vi "Utilisation des boucles.vi"() -> ()   [LabVIEW 2017]
panel:
  in  "V end":dbl format="%#_13g"
  in  "V0":dbl format="%#_13g"
  out "Waveform Graph 2":dbl[](graph)
  in  "Step":dbl format="%#_13g"
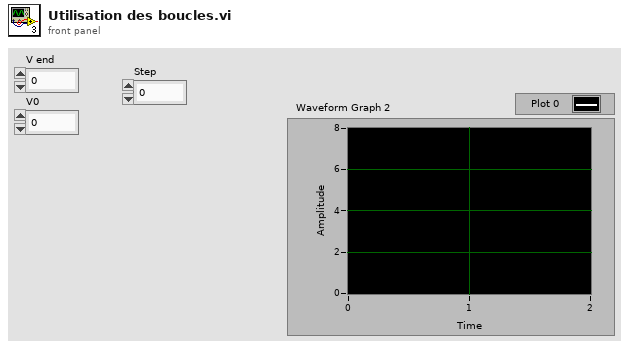
[diagram p1: front panel]
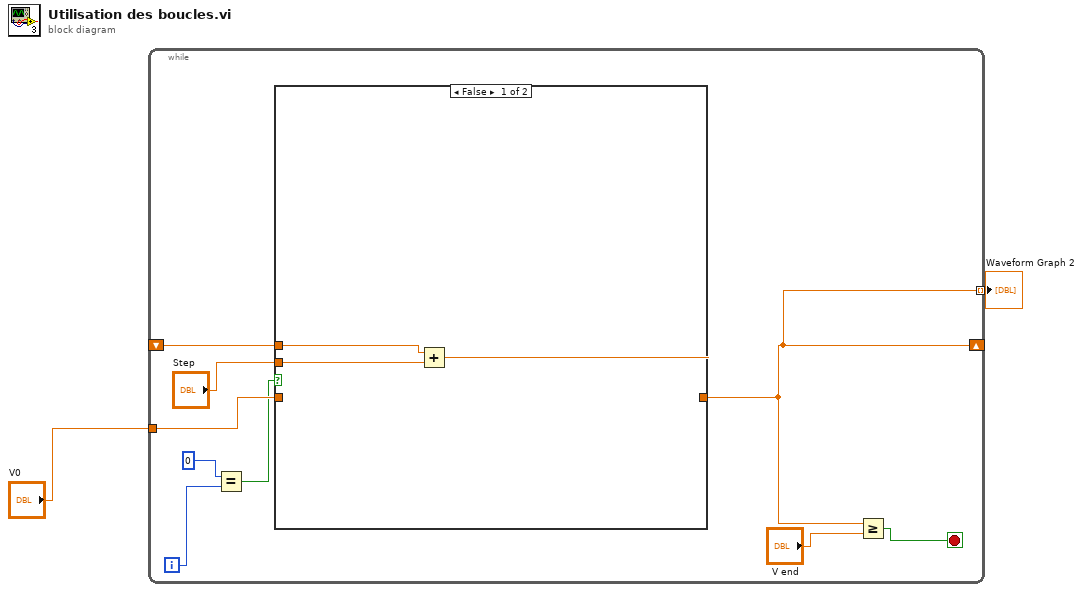
[diagram p0: block diagram]
diagram:
  n1 = while {
    tunnel: "V0" -> [w11]
    shift-right: [w4] -> _
    shift-left: _ -> [w7]
    tunnel: [w4] -> w1 mode=indexing
    i -> [w8]
    stop <- w3 stop-if-true
    n2 = Equal?(x=0, y=w8) -> (x = y?=w10:bool)
    n3 = case shown="False" w10 {
      tunnel: [w12 w15] -> w4
      tunnel: w11 -> [_ w15]
      tunnel: w7 -> [w14 _]
      tunnel: "Step" -> [w13 _]
      frame False {
        n4 = Add(x=w14, y=w13) -> (x+y=w12:dbl)
      }
      frame True {
      }
    }
    n5 = Greater Or Equal?(x=w4, y="V end") -> (x >= y?=w3:bool)
  }
  "Waveform Graph 2" <- w1
